vi "Drone video to IMAQ - Main (SubVI).vi"() -> (0 "error out":errorcluster, 1 "Video Stream":picture, 2 "new picture":picture, 3 "Refnum out":T1)   [LabVIEW 2014]
uses:
  <vilib>/vision/Image Controls.llb/IMAQ Image.ctl
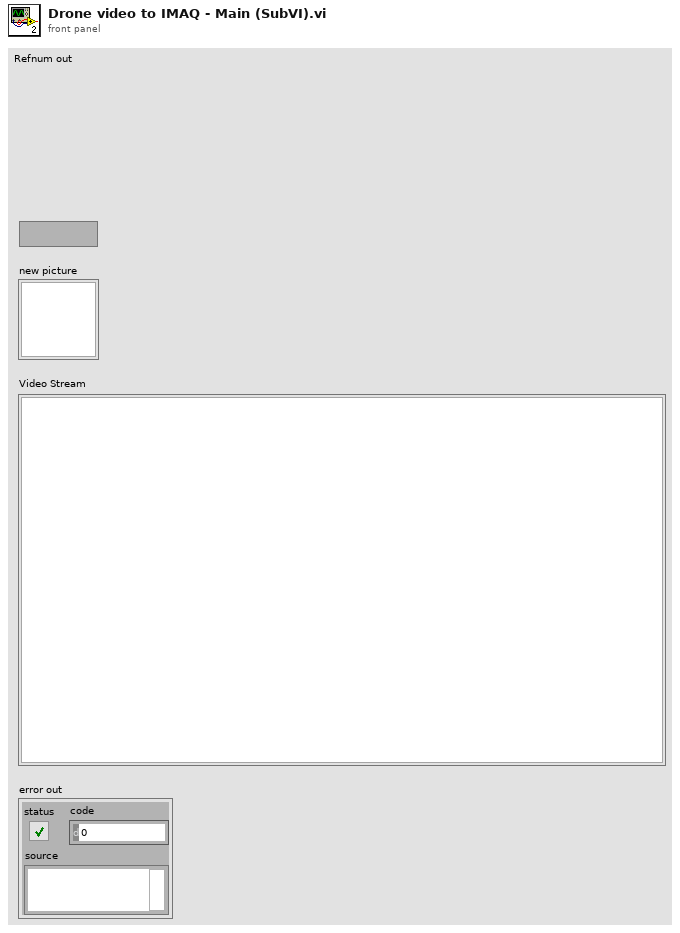
[diagram p1: front panel]
types:
  T1 = typedef "IMAQ Image.ctl" = refnum<image>
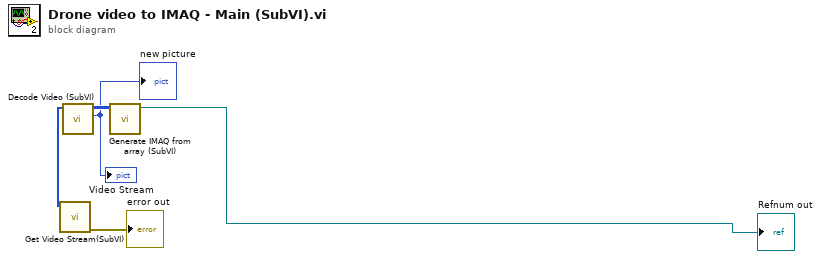
[diagram p0: block diagram]
diagram:
  n1 = call "Get Video Stream(SubVI).vi"() -> ("error out"=→"error out":errorcluster, "ImgData"=w1:u8[])  [unwired: 10 in]
  n2 = call "Decode Video (SubVI).vi"("ImgData"=w1) -> ("new picture"=→"Video Stream" →"new picture":picture, "Array"=w3:u32[][])  [unwired: 9 in]
  n3 = call "Generate IMAQ from array (SubVI).vi"("Array"=w3) -> ("Refnum out"=→"Refnum out":T1)  [unwired: 10 in]
